vi "Camera Command Handle.vi"(4 "Value":string, 6 "Var Name":string, 8 "error in (no error)":errorcluster, 9 "String":string, 10 "command":string, 11 "connection ID":refnum<k5>) -> (0 "error out":errorcluster, 2 "Command Accepted":bool, 3 "connection ID 2":refnum<k5>)   [LabVIEW 2024, in "cameraV1.lvlib"]
uses:
  cameraV1.lvlib
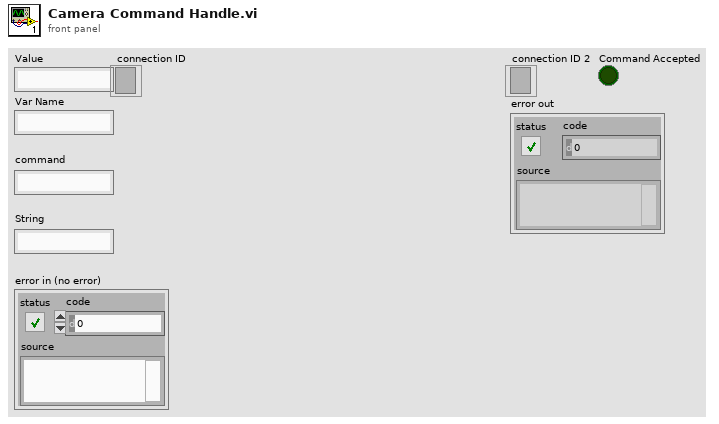
[diagram p1: front panel]
types:
  T1 = enum16{"Standard", "Buffered", "CRLF", "Immediate"}
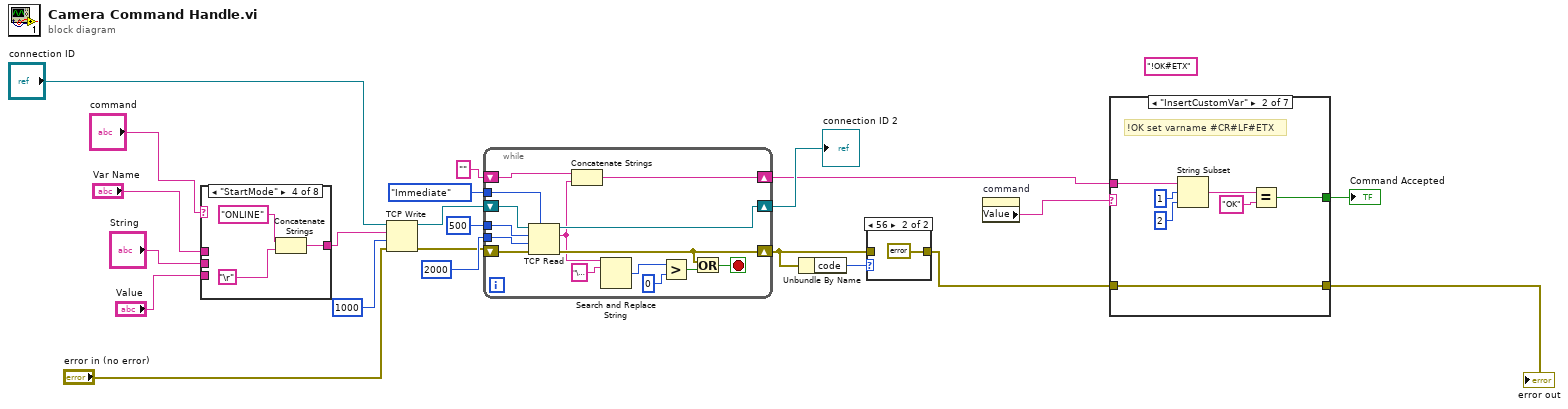
[diagram p0: block diagram]
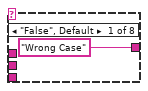
[diagram p2: hidden frame]
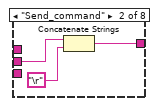
[diagram p3: hidden frame]
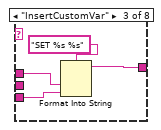
[diagram p4: hidden frame]
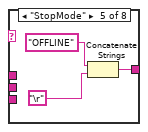
[diagram p5: hidden frame]
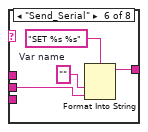
[diagram p6: hidden frame]
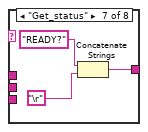
[diagram p7: hidden frame]
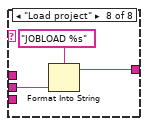
[diagram p8: hidden frame]
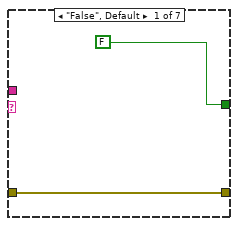
[diagram p9: hidden frame]
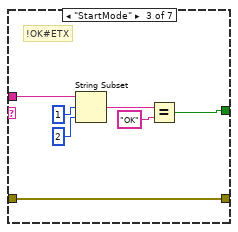
[diagram p10: hidden frame]
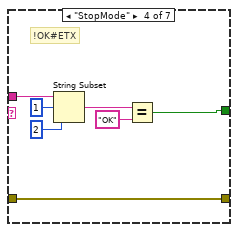
[diagram p11: hidden frame]
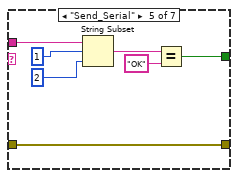
[diagram p12: hidden frame]
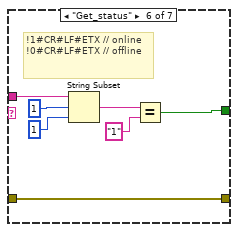
[diagram p13: hidden frame]
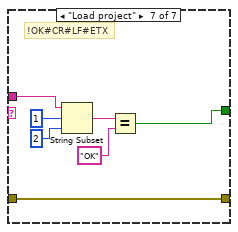
[diagram p14: hidden frame]
diagram:
  (unwired) "!OK#ETX" ("format string")
  n1 = case shown="\"StartMode\"" "command" {
    tunnel: "String" -> [_ w25 _ _ _ w37 _ w45]
    tunnel: ["Wrong Case" w24 w27 w31 w35 w40 w41 w44] -> w4
    tunnel: "Var Name" -> [_ _ w29 _ _ _ _ _]
    tunnel: "Value" -> [_ _ w28 _ _ _ _ _]
    frame "False", Default {
    }
    frame "Send_command" {
      n2 = Concatenate Strings(w25, "\r") -> (w24:string)
    }
    frame "InsertCustomVar" {
      n3 = Format Into String(format string="SET %s %s" ("Command"), w29, w28) -> (resulting string=w27:string)  [unwired: 2 in, 1 out]
    }
    frame "StartMode" {
      n4 = Concatenate Strings("ONLINE" ("Command"), "\r") -> (w31:string)
    }
    frame "StopMode" {
      n5 = Concatenate Strings("OFFLINE" ("Command"), "\r") -> (w35:string)
    }
    frame "Send_Serial" {
      w38 = ""  # Var name
      n6 = Format Into String(format string="SET %s %s" ("Command"), w38, w37) -> (resulting string=w40:string)  [unwired: 2 in, 1 out]
    }
    frame "Get_status" {
      n7 = Concatenate Strings("READY?" ("Command"), "\r") -> (w41:string)
    }
    frame "Load project" {
      n8 = Format Into String(format string="JOBLOAD %s" ("Command"), w45) -> (resulting string=w44:string)  [unwired: 2 in, 1 out]
    }
  }
  n9 = TCP Write(connection ID="connection ID", data in=w4, error in (no error)="error in (no error)", 9:1000 ("timeout ms (25000)")) -> (connection ID out=w16:refnum<k5>, error out=w10:errorcluster)  [unwired: 1 out]
  n10 = while {
    tunnel: T1."Immediate" ("mode (standard)") -> [w60]
    tunnel: 2000 ("timeout ms (25000)") -> [w59]
    tunnel: 500 ("bytes to read") -> [w56]
    shift-right: [w57] -> w15
    shift-left: w16 -> [w61]
    shift-right: [w52] -> w13
    shift-left: w10 -> [w58]
    shift-right: [w55] -> w11
    shift-left: "" -> [w54]
    stop <- w53 stop-if-true
    n11 = TCP Read(connection ID=w61, bytes to read=w56, error in (no error)=w58, 7:w60, 9:w59) -> (connection ID out=w57:refnum<k5>, data out=w50:string, error out=w52:errorcluster)
    n12 = Concatenate Strings(w54, w50) -> (w55:string)
    n13 = Search and Replace String(input string=w50, search string="\u0003" ("y")) -> (number of replacements=w49:i32)  [unwired: 6 in, 3 out]
    n14 = Greater?(x=w49, y=0) -> (0:w48:bool)
    n15 = Or(x=w52, y=w48) -> (x .or. y?=w53:bool)
  }
  "connection ID 2" <- w15
  n16 = Unbundle By Name(w13) -> ("code"=w14:i32)
  n17 = case shown="56" w14 {
    tunnel: [w62 errorcluster {"status"=FALSE, "code"=0, "source"=""} ("error out")] -> w1
    tunnel: w13 -> [w62 _]
    frame 0, Default {
    }
    frame 56 {
    }
  }
  n18 = property on="command" class="Str"() -> ("Value"=w3:string)  [unwired: 2 in, 2 out]
  n19 = case shown="\"InsertCustomVar\"" w3 {
    tunnel: w11 -> [_ w69 w77 w84 w89 w95 w105]
    tunnel: [FALSE w70 w78 w85 w88 w99 w106] -> w12
    tunnel: [w64 w66 w73 w80 w87 w94 w101] -> w2
    tunnel: w1 -> [w64 w66 w73 w80 w87 w94 w101]
    frame "False", Default {
    }
    frame "InsertCustomVar" {
      # "!OK set varname #CR#LF#ETX"
      n20 = String Subset(string=w69, offset (0)=1, length (rest)=2 ("y")) -> (substring=w67:string)
      n21 = Equal?(x=w67, y="OK" ("format string")) -> (x = y?=w70:bool)
    }
    frame "StartMode" {
      # "!OK#ETX"
      n22 = String Subset(string=w77, offset (0)=1, length (rest)=2 ("y")) -> (substring=w74:string)
      n23 = Equal?(x=w74, y="OK" ("format string")) -> (x = y?=w78:bool)
    }
    frame "StopMode" {
      # "!OK#ETX"
      n24 = String Subset(string=w84, offset (0)=1, length (rest)=2 ("y")) -> (substring=w81:string)
      n25 = Equal?(x=w81, y="OK" ("format string")) -> (x = y?=w85:bool)
    }
    frame "Send_Serial" {
      n26 = String Subset(string=w89, offset (0)=1, length (rest)=2 ("y")) -> (substring=w93:string)
      n27 = Equal?(x=w93, y="OK" ("format string")) -> (x = y?=w88:bool)
    }
    frame "Get_status" {
      # "!1#CR#LF#ETX // online\n!0#CR#LF#ETX // offline"
      n28 = String Subset(string=w95, offset (0)=1, length (rest)=1 ("y")) -> (substring=w98:string)
      n29 = Equal?(x=w98, y="1" ("format string")) -> (x = y?=w99:bool)
    }
    frame "Load project" {
      # "!OK#CR#LF#ETX"
      n30 = String Subset(string=w105, offset (0)=1, length (rest)=2 ("offset (0)")) -> (substring=w104:string)
      n31 = Equal?(x=w104, y="OK" ("format string")) -> (x = y?=w106:bool)
    }
  }
  "error out" <- w2
  "Command Accepted" <- w12
